vi "Synth Reset.vi"(8 "Error In":errorcluster, 11 "DAQmx Device Name":tag) -> (0 "Error Out":errorcluster, 3 "DAQmx Device Name out":tag)   [LabVIEW 2015]
uses:
  <vilib>/DAQmx/write.llb/DAQmx Write (Digital Bool 1Line 1Point).vi
  <vilib>/DAQmx/create/channels.llb/DAQmx Create Channel (DO-Digital Output).vi
  <vilib>/DAQmx/miscellaneous.llb/DAQmx Fill In Error Info.vi
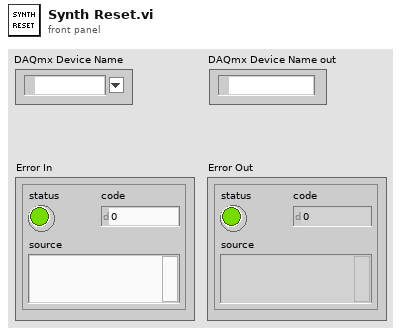
[diagram p1: front panel]
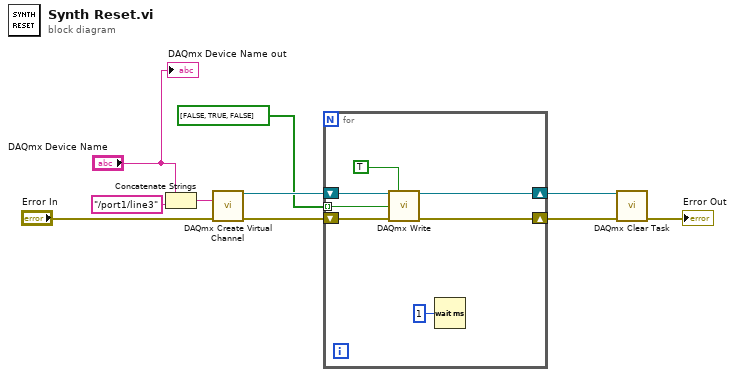
[diagram p0: block diagram]
diagram:
  n1 = Concatenate Strings("DAQmx Device Name", "/port1/line3") -> (w5:string)
  n2 = call-poly <vilib>:"DAQmx Create Virtual Channel.vi"("lines"=w5, "error in"="Error In") -> ("task out"=w9:refnum<k21>, "error out"=w10:errorcluster)  [unwired: 3 in, 9 out]
  n3 = for {
    shift-right: [w15] -> w6
    shift-left: w10 -> [w17]
    shift-right: [w14] -> w8
    shift-left: w9 -> [w16]
    tunnel: bool[] [FALSE, TRUE, FALSE] -> [w11] mode=indexing
    n4 = call-poly <vilib>:"DAQmx Write.vi"("task/channels in"=w16, "auto start"=TRUE, "data"=w11, "error in"=w17) -> ("task out"=w14:refnum<k21>, "error out"=w15:errorcluster)  [unwired: 10 out]
    n5 = Wait (ms)(milliseconds to wait=u32 1) -> ()  [unwired: 1 out]
  }
  n6 = call <vilib>:"DAQmx Clear Task.vi"("task in"=w8, "error in"=w6) -> ("error out"=→"Error Out":errorcluster)  [unwired: 13 out]
  "DAQmx Device Name out" <- "DAQmx Device Name"
